vi "XY Fit.vi"(0 "Outlier Cutoff":dbl=3.0, 5 "X Values":dbl[](array[numeric]), 7 "Y Values":dbl[](array[numeric])) -> (4 "slope":dbl, 6 "intercept":dbl, 8 "R-square":dbl, 10 "mean":dbl, 14 "XY Graph":cluster{dbl[], dbl[]}[](graph))   [LabVIEW 2013]
uses:
  <vilib>/Analysis/baseanly.llb/Mean (DBL).vi
  <vilib>/Analysis/NI_AALPro.lvlib
  <vilib>/Analysis/NI_AALBase.lvlib
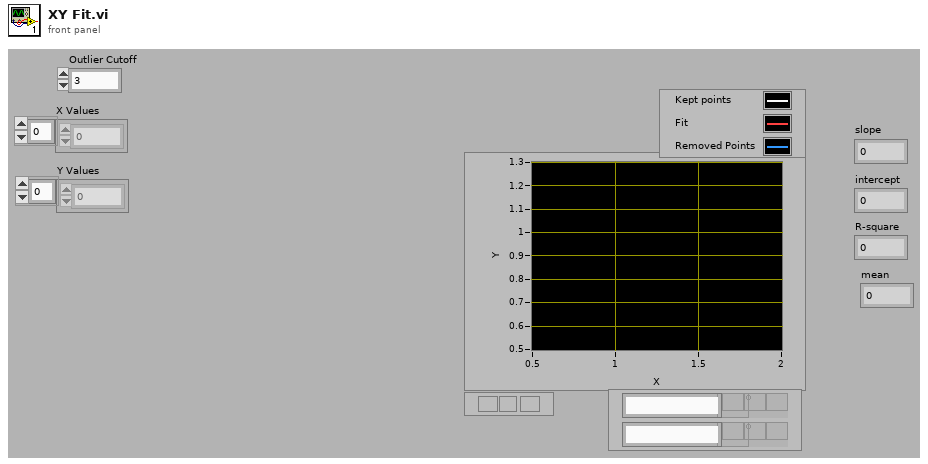
[diagram p1: front panel]
types:
  T1 = cluster{"X Values":dbl[], "Best Linear Fit":dbl[]}
  T2 = cluster{"X Values":dbl[], "Best Linear Fit":dbl[]}[]
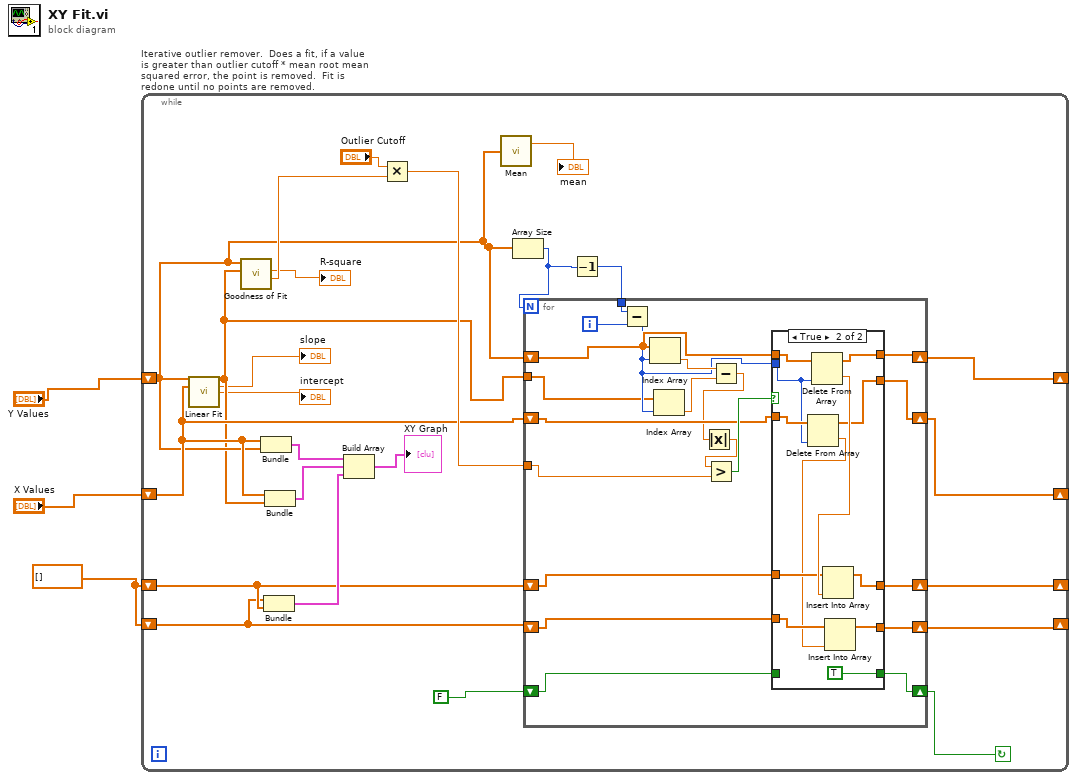
[diagram p0: block diagram]
diagram:
  w1 = dbl[] []
  n1 = while "Iterative outlier remover.  Does a fit, if a value is greater than outlier cutoff * mean root mean squared error, the point is removed.  Fit is redone until no points are removed." {
    shift-right: [w18] -> _
    shift-left: "Y Values" -> [w10]
    shift-right: [w19] -> _
    shift-left: "X Values" -> [w14]
    shift-right: [w20] -> _
    shift-left: w1 -> [w12]
    shift-right: [w17] -> _
    shift-left: w1 -> [w11]
    stop <- w15 continue-if-true
    n2 = call <vilib>:"Linear Fit.vi"("Y"=w10, "X"=w14) -> ("Best Linear Fit"=w9:dbl[], "slope"=→"slope":dbl, "intercept"=→"intercept":dbl)  [unwired: 9 in, 2 out]
    n3 = call <vilib>:"Goodness of Fit.vi"("Best Fit"=w9, "Y"=w10) -> ("RMSE"=w24:dbl, "R-square"=→"R-square":dbl)  [unwired: 6 in, 2 out]
    n4 = Bundle("X Values"=w14, "Y Values"=w10) -> (w27:cluster{"X Values":dbl[], "Y Values":dbl[]})  [unwired: 1 in]
    n5 = Bundle(w11, w12) -> (w13:cluster{dbl[], dbl[]})  [unwired: 1 in]
    n6 = Bundle("X Values"=w14, "Best Linear Fit"=w9) -> (w25:T1)  [unwired: 1 in]
    n7 = Build Array(w27, w25, w13) -> (→"XY Graph":T2)
    n8 = Multiply(x="Outlier Cutoff", y=w24) -> (x*y=w23:dbl)
    n9 = call-poly <vilib>:"Mean.vi"("X"=w10) -> ("mean"=→"mean":dbl)  [unwired: 1 out]
    n10 = Array Size(array=w10) -> (size(s)=w22:i32)
    n11 = Decrement(x=w22) -> (x-1=w21:i32)
    n12 = for {
      N: w22 -> [_]
      tunnel: w23 -> [w47]
      tunnel: w21 -> [w45]
      shift-right: [w41] -> w19
      shift-left: w14 -> [w30]
      shift-right: [w39] -> w18
      shift-left: w10 -> [w40]
      shift-right: [w36] -> w20
      shift-left: w12 -> [w37]
      shift-right: [w34] -> w17
      shift-left: w11 -> [w35]
      shift-right: [w33] -> w15
      shift-left: FALSE -> [w32]
      tunnel: w9 -> [w31]
      i -> [w46]
      n13 = Subtract(x=w45, y=w46) -> (x-y=w38:i32)
      n14 = Index Array(array=w40, index=w38) -> (element=w44:dbl)
      n15 = Index Array(array=w31, index=w38) -> (element=w43:dbl)
      n16 = Subtract(x=w44, y=w43) -> (x-y=w29:dbl)
      n17 = Absolute Value(x=w29) -> (abs(x)=w28:dbl)
      n18 = Greater?(x=w28, y=w47) -> (0:w42:bool)
      n19 = case shown="True" w42 {
        tunnel: w30 -> [w52 w59]
        tunnel: [w52 w57] -> w41
        tunnel: w40 -> [w51 w64]
        tunnel: [w51 w63] -> w39
        tunnel: w38 -> [_ w58]
        tunnel: w37 -> [w50 w61]
        tunnel: [w50 w60] -> w36
        tunnel: w35 -> [w49 w56]
        tunnel: [w49 w55] -> w34
        tunnel: [w48 TRUE] -> w33
        tunnel: w32 -> [w48 _]
        frame False {
        }
        frame True {
          n20 = Delete From Array(array=w59, index=w58) -> (deleted portion=w54:dbl, array with subset deleted=w57:dbl[])  [unwired: 1 in]
          n21 = Delete From Array(array=w64, index=w58) -> (deleted portion=w62:dbl, array with subset deleted=w63:dbl[])  [unwired: 1 in]
          n22 = Insert Into Array(array=w61, new element=w62) -> (w60:dbl[])  [unwired: 1 in]
          n23 = Insert Into Array(array=w56, new element=w54) -> (w55:dbl[])  [unwired: 1 in]
        }
      }
    }
  }
